vi "Module Top Level.vi"(8 "error in":errorcluster) -> (0 "error out":errorcluster)   [LabVIEW 2018, in "PC UDP Reader.lvlib"]
doc: "This is the top level VI for this module. It uses a queue for communications and is stopped user a user event. The general architecture is similar to a simple queued message handler.\n\nThe VIs associated with this module are organized in a LabVIEW Library."
uses:
  PC UDP Reader.lvlib
  Private Controls/cRIO RT Comms Data.ctl
  Private Controls/Module Data.ctl
  Private Controls/Module Action.ctl
  Top Level/Shared Controls/All Data Cluster.ctl
  Top Level/Shared Controls/Acq Data.ctl
  Globals/Host Globals.vi
  Error Handler/Error Handler.lvlib
  Controller (Host)/Controller (Host).lvlib
panel:
  out "Connected?":bool
  # "UDP Reader"
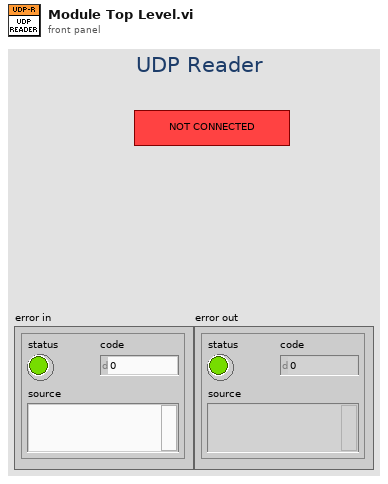
[diagram p1: front panel]
types:
  T1 = typedef "PC UDP Reader.lvlib/cRIO RT Comms Data.ctl" = cluster{"Connected?":bool, "connection ID":refnum<k16>}
  T2 = typedef "PC UDP Reader.lvlib/Module Data.ctl" = cluster{"Data":variant, "Action":T3}
  T3 = typedef "PC UDP Reader.lvlib/Module Action.ctl" = enum8{"Init", "Read", "Error", "Exit"}
  T4 = typedef "All Data Cluster.ctl" = cluster{"AI":T5, "Accel Data":cluster{"Accel RMS(in/sec2)":dbl[], "Accel Peak(in/sec2)":dbl[], "Velocity RMS(in/sec)":dbl[], "Velocity Peak(in/sec)":dbl[]}, "Temps":cluster{"01-00-9213":dbl[], "01-01-9213":dbl[], "01-02-9213":dbl[]}, "00-03-9402(RPM)":dbl[], "02-04-9871":dbl[], "ARINC":sgl[]}
  T5 = typedef "Acq Data.ctl" = cluster{"00-00-9220":dbl[], "00-01-9220":dbl[], "02-02-9219":dbl[], "02-03-9227":dbl[], "02-05-9205":dbl[]}
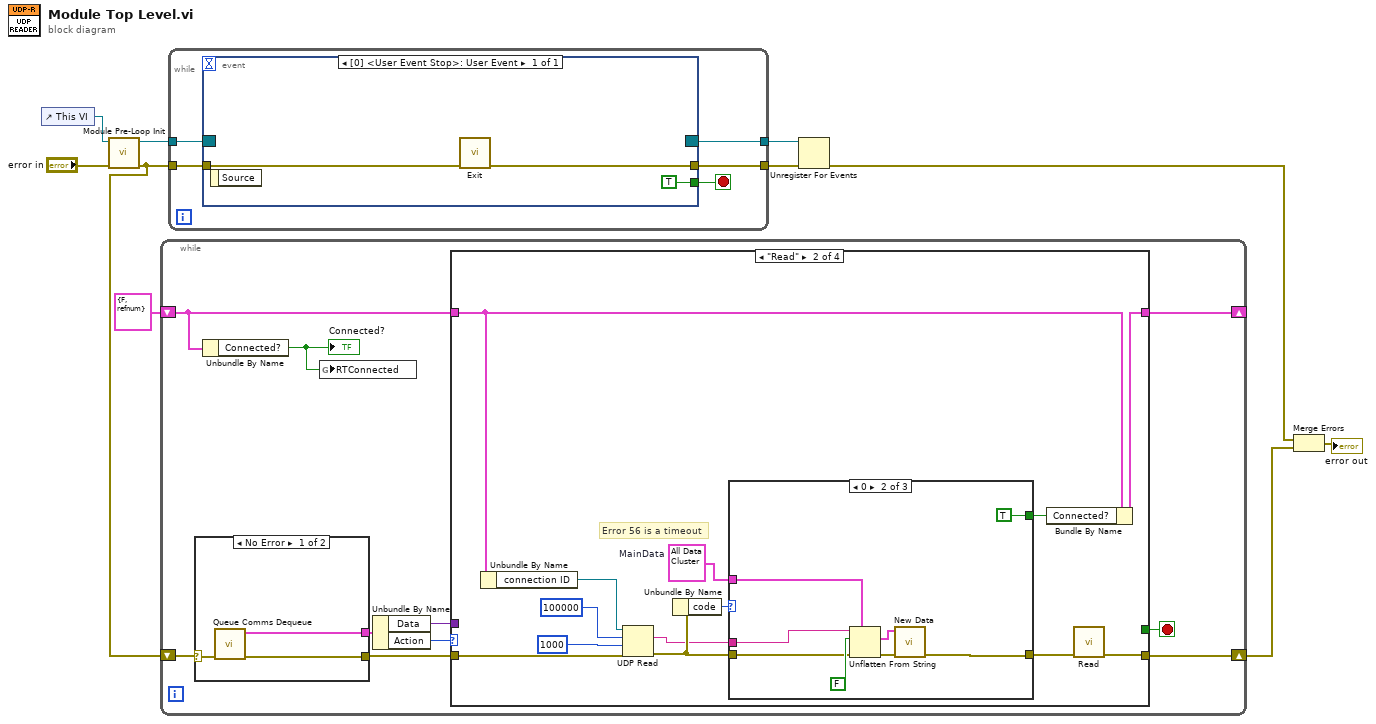
[diagram p0: block diagram]
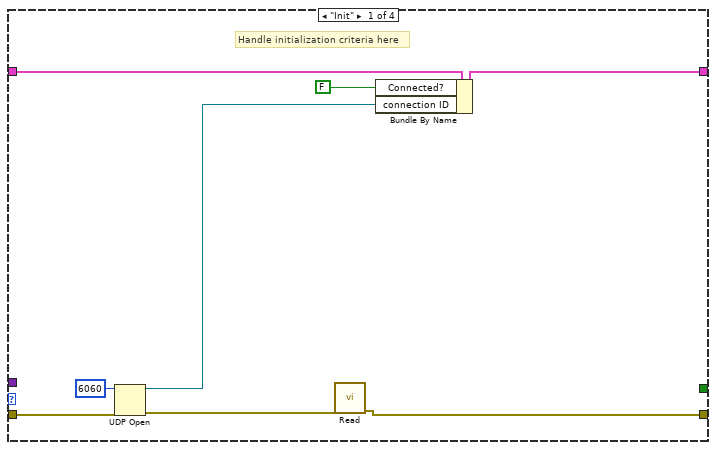
[diagram p2: hidden frame]
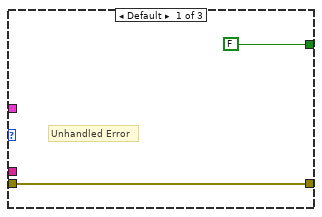
[diagram p3: hidden frame]
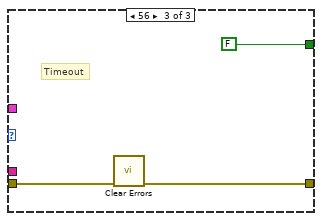
[diagram p4: hidden frame]
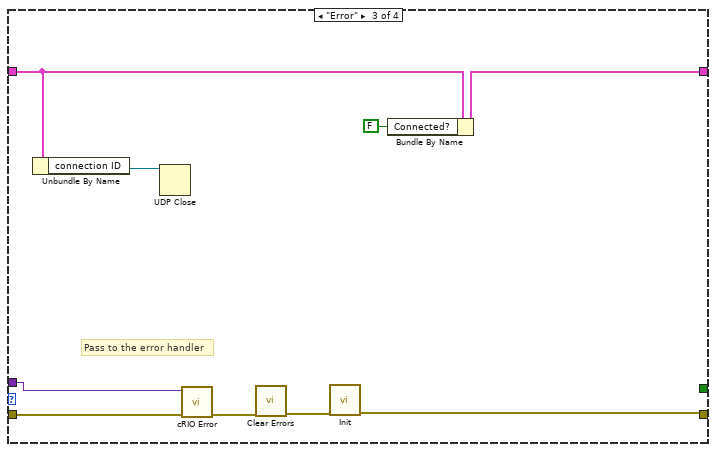
[diagram p5: hidden frame]
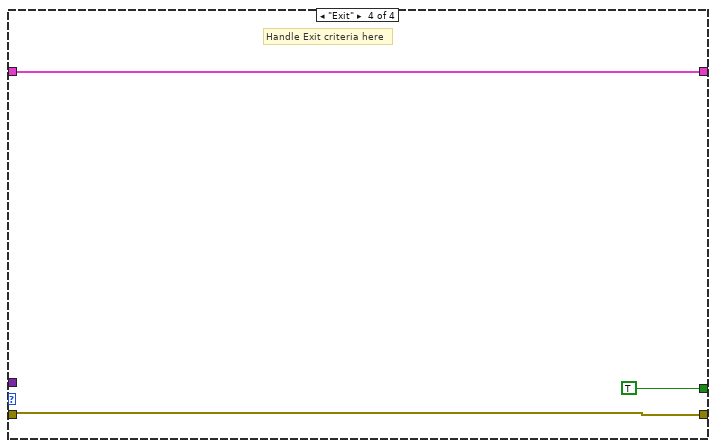
[diagram p6: hidden frame]
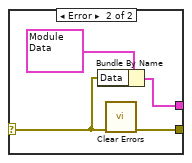
[diagram p7: hidden frame]
diagram:
  n1 = control-ref of="This VI"() -> (w10:refnum<vi>)
  n2 = call "Module Pre-Loop Init.vi"("error in (no error)"="error in", "Top Level VI Ref in"=w10) -> ("error out"=w3:errorcluster, "User Event Stop Ref"=w9:refnum<event-registration>)  [unwired: 8 in]
  n3 = while {
    shift-right: [w15] -> w6
    shift-left: w3 -> [w14]
    shift-right: [w13] -> _
    shift-left: T1 {"Connected?"=FALSE, "connection ID"=refnum} ("cRIO RT Comms Data out") -> [w12]
    stop <- w16 stop-if-true
    n4 = case shown="No Error" w14 {
      selector: w14 -> [w68 w71]
      tunnel: [w69 w72] -> w20
      tunnel: [w67 w70] -> w17
      frame No Error {
        n5 = call "Queue Comms Dequeue.vi"("error in (no error)"=w68) -> ("error out"=w67:errorcluster, "element"=w69:T2)  [unwired: 8 in, 1 out]
      }
      frame Error {
        n6 = Bundle By Name(cluster=T2 {"Data"=variant, "Action"=enum."Error"} ("element"), "Data"=w71) -> (w72:T2)
        n7 = call <vilib>:"Clear Errors.vi"("error in (no error)"=w71) -> ("error out"=w70:errorcluster)  [unwired: 5 in, 1 out]
      }
    }
    n8 = Unbundle By Name(w12) -> ("Connected?"=w11:bool)
    "Connected?" <- w11
    n9 = global write "Host Globals.vi" "RTConnected"(w11) -> ()
    n10 = Unbundle By Name(w20) -> ("Data"=w18:variant, "Action"=w19:T3)
    n11 = case shown="\"Read\"" w19 {
      tunnel: w18 -> [_ _ w62 _]
      tunnel: w17 -> [w25 w39 w63 w64]
      tunnel: [w21 w36 w55 w64] -> w15
      tunnel: [_ _ _ TRUE] -> w16
      tunnel: w12 -> [w28 w41 w59 w65]
      tunnel: [w27 w35 w61 w65] -> w13
      frame "Init" {
        # "Handle initialization criteria here"
        n12 = UDP Open(8:w25, 11:u16 6060 ("port")) -> (port=w23:refnum<k16>, 0:w22:errorcluster)  [unwired: 3 in, 1 out]
        n13 = call "Read.vi"("error in"=w22) -> ("error out"=w21:errorcluster)  [unwired: 10 in]
        n14 = Bundle By Name(cluster=w28, "Connected?"=FALSE, "connection ID"=w23) -> (w27:T1)
      }
      frame "Read" {
        w29 = T4 {"AI"={"00-00-9220"=[], "00-01-9220"=[], "02-02-9219"=[], "02-03-9227"=[], "02-05-9205"=[]}, "Accel Data"={"Accel RMS(in/sec2)"=[], "Accel Peak(in/sec2)"=[], "Velocity RMS(in/sec)"=[], "Velocity Peak(in/sec)"=[]}, "Temps"={"01-00-9213"=[], "01-01-9213"=[], "01-02-9213"=[]}, "00-03-9402(RPM)"=[], "02-04-9871"=[], "ARINC"=[]}  # MainData
        # "Error 56 is a timeout"
        n15 = Unbundle By Name(w41) -> ("connection ID"=w40:refnum<k16>)
        n16 = UDP Read(connection ID=w40, max size (548)=100000, timeout ms (25000)=1000, 8:w39) -> (data out=w30:string, error out=w33:errorcluster)  [unwired: 3 out]
        n17 = Unbundle By Name(w33) -> ("code"=w32:i32)
        n18 = case shown="0" w32 {
          tunnel: [w43 w50 w52] -> w37
          tunnel: w30 -> [_ w49 _]
          tunnel: [FALSE TRUE FALSE] -> w34
          tunnel: w33 -> [w43 w47 w54]
          tunnel: w29 -> [_ w46 _]
          frame Default {
            # "Unhandled Error"
          }
          frame 0 {
            n19 = Unflatten From String(type=w46, binary string=w49, data includes array or string size? (T)=FALSE, error in (no error)=w47) -> (value=w45:T4, error out=w44:errorcluster)  [unwired: 1 in, 1 out]
            n20 = call "New Data.vi"("error in"=w44, "cRIOData"=w45) -> ("error out"=w50:errorcluster)  [unwired: 9 in]
          }
          frame 56 {
            # "Timeout"
            n21 = call <vilib>:"Clear Errors.vi"("error in (no error)"=w54) -> ("error out"=w52:errorcluster)  [unwired: 5 in, 1 out]
          }
        }
        n22 = Bundle By Name(cluster=w41, "Connected?"=w34) -> (w35:T1)
        n23 = call "Read.vi"("error in"=w37) -> ("error out"=w36:errorcluster)  [unwired: 10 in]
      }
      frame "Error" {
        # "Pass to the error handler"
        n24 = Unbundle By Name(w59) -> ("connection ID"=w58:refnum<k16>)
        n25 = UDP Close(connection ID=w58) -> ()  [unwired: 1 in, 2 out]
        n26 = call "cRIO Error.vi"("error in (no error)"=w63, "Data"=w62) -> ("error out"=w57:errorcluster)  [unwired: 9 in]
        n27 = call <vilib>:"Clear Errors.vi"("error in (no error)"=w57) -> ("error out"=w56:errorcluster)  [unwired: 5 in, 1 out]
        n28 = call "Init.vi"("error in"=w56) -> ("error out"=w55:errorcluster)  [unwired: 10 in]
        n29 = Bundle By Name(cluster=w59, "Connected?"=FALSE) -> (w61:T1)
      }
      frame "Exit" {
        # "Handle Exit criteria here"
      }
    }
  }
  n30 = while {
    tunnel: w9 -> [w78]
    tunnel: [w77] -> w7
    tunnel: w3 -> [w76]
    tunnel: [w74] -> w8
    stop <- w75 stop-if-true
    n31 = event shown="[0] <User Event Stop>: User Event" {
      selector: w78 -> [_]
      dyn-events: [_] -> w74
      timeout: _ -> [_]
      tunnel: [w79] -> w77
      tunnel: w76 -> [w80]
      tunnel: [TRUE] -> w75
      event User Event {
        n32 = event-data() -> ()  [unwired: 1 in, 1 out]
        n33 = call "Exit.vi"("error in (no error)"=w80) -> ("error out"=w79:errorcluster)  [unwired: 10 in]
      }
    }
  }
  n34 = Unregister For Events(event registration refnum=w8, error in=w7) -> (error out=w5:errorcluster)
  n35 = Merge Errors(w5, w6) -> (→"error out":errorcluster)
